vi "WritePATH.vi"(8 "error in (no error)":errorcluster, 10 "Path":path, 11 "Loggin in":refnum<class "Loggin.lvclass">) -> (0 "error out":errorcluster, 3 "Loggin out":refnum<class "Loggin.lvclass">)   [LabVIEW 2020, in "Loggin.lvlib" / "Loggin.lvclass"]
uses:
  Loggin.lvclass
  Loggin.lvclass/Loggin.ctl
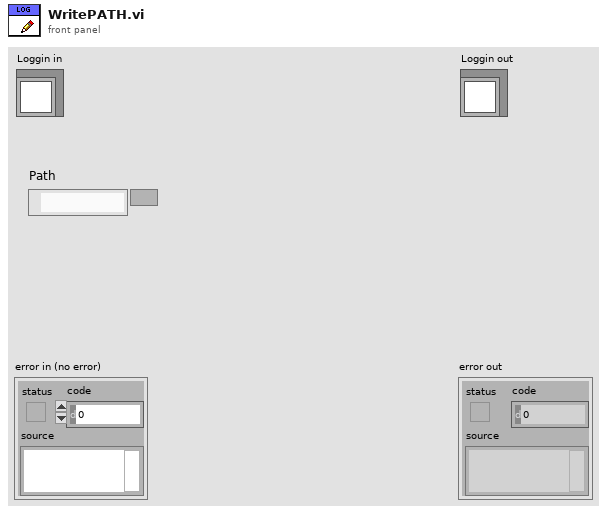
[diagram p1: front panel]
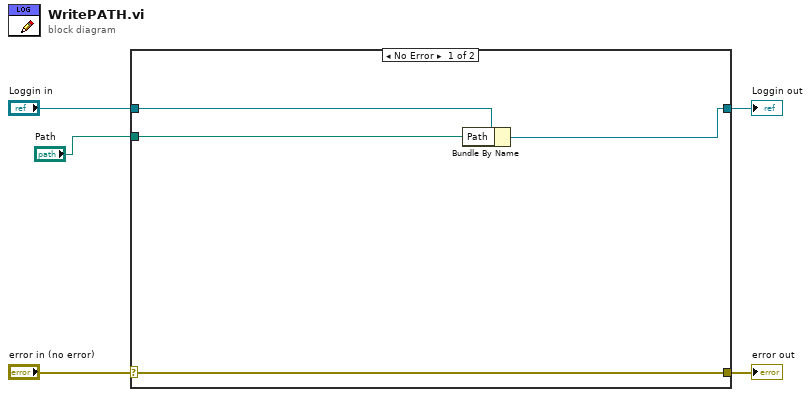
[diagram p0: block diagram]
diagram:
  n1 = case shown="No Error" "error in (no error)" {
    selector: "error in (no error)" -> [w9 w11]
    tunnel: [w9 w11] -> w4
    tunnel: [w7 w10] -> w2
    tunnel: "Loggin in" -> [w8 w10]
    tunnel: "Path" -> [w6 _]
    frame No Error {
      n2 = Bundle By Name(cluster=w8, "Path"=w6) -> (w7:refnum<class "Loggin.lvclass">)
    }
    frame Error {
    }
  }
  "error out" <- w4
  "Loggin out" <- w2
